vi "按钮sin2.vi"() -> ()   [LabVIEW 2018]
panel:
  in  "停止":bool
  in  "确定按钮":bool
  out "布尔":bool
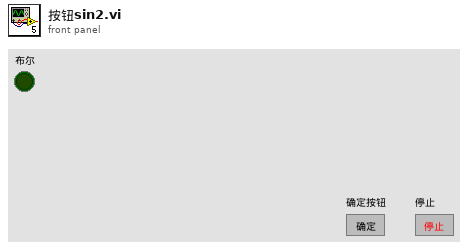
[diagram p1: front panel]
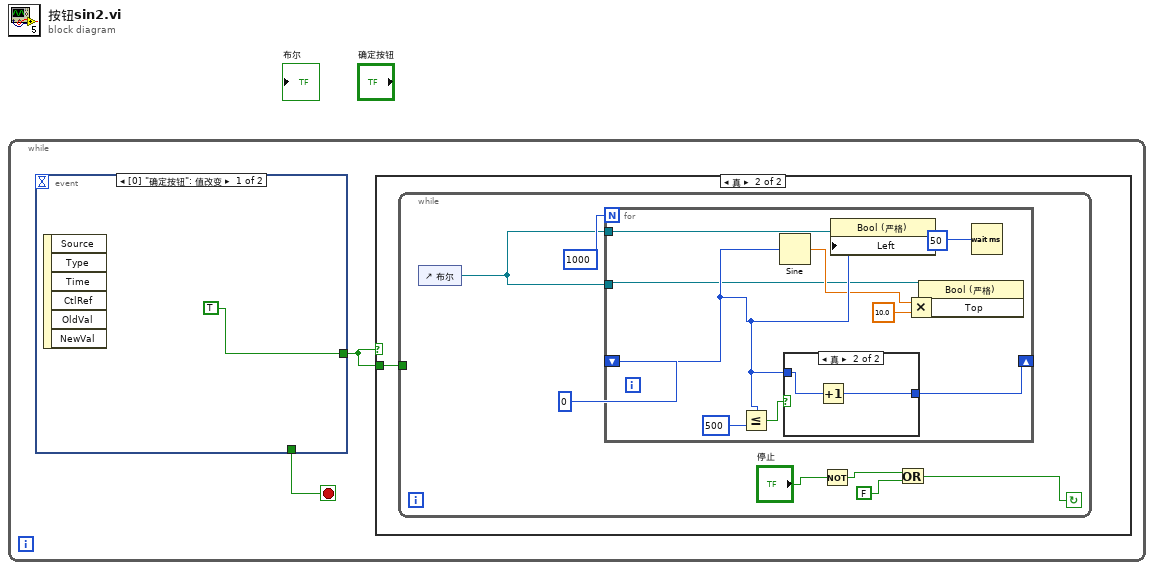
[diagram p0: block diagram]
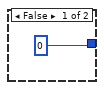
[diagram p3: hidden frame]
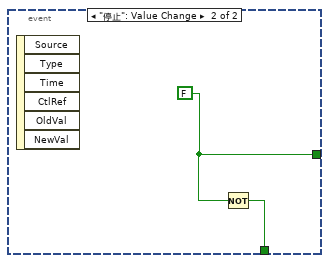
[diagram p4: hidden frame]
diagram:
  n1 = while {
    stop <- w2 stop-if-true
    n2 = event shown="[0] \"确定按钮\": 值改变" {
      selector: _ -> [_ _]
      dyn-events: _ -> [_ _]
      timeout: _ -> [_ _]
      tunnel: [TRUE w26] -> w1
      tunnel: [_ w25] -> w2
      event "确定按钮": Value Change {
        n3 = event-data() -> ()  [unwired: 1 in, 6 out]
      }
      event "停止": Value Change {
        w26 = FALSE
        n4 = event-data() -> ()  [unwired: 1 in, 6 out]
        n5 = Not(x=w26) -> (.not. x?=w25:bool)
      }
    }
    n6 = case shown="真" w1 {
      tunnel: w1 -> [_ w3]
      frame False {
      }
      frame True {
        n7 = while {
          tunnel: w3 -> [_]
          stop <- w6 continue-if-true
          n8 = control-ref of="布尔"() -> (w8:refnum<vi>)
          n9 = for {
            N: 1000 -> [_]
            shift-right: [w18] -> _
            shift-left: 0 -> [w17]
            tunnel: w8 -> [w12]
            tunnel: w8 -> [w11]
            n10 = Less Or Equal?(x=w17, y=500) -> (x <= y?=w20:bool)
            n11 = Sine(x=w17) -> (sin(x)=w15:dbl)
            n12 = case shown="真" w20 {
              tunnel: w17 -> [_ w23]
              tunnel: [0 w22] -> w18
              frame False {
              }
              frame True {
                n13 = Increment(x=w23) -> (x+1=w22:i32)
              }
            }
            n14 = property on="属性节点" class="Bool (严格)"(reference=w12, "Left"=w17) -> ()  [unwired: 1 in, 2 out]
            n15 = Multiply(x=w15, y=10.0) -> (x*y=w14:dbl)
            n16 = property on="属性节点" class="Bool (严格)"(reference=w11, "Top"=w14) -> ()  [unwired: 1 in, 2 out]
            n17 = Wait (ms)(milliseconds to wait=u32 50 ("等待时间（毫秒）")) -> ()  [unwired: 1 out]
          }
          n18 = Not(x="停止") -> (.not. x?=w4:bool)
          n19 = Or(x=w4, y=FALSE) -> (x .or. y?=w6:bool)
        }
      }
    }
  }
